vi "Read decimation factors.vi"(8 "error in (no error)":errorcluster, 11 "Runtime.Transfer in":refnum<class "Runtime.Transfer.lvclass">) -> (0 "error out":errorcluster, 2 "decimation factors":T1, 3 "Runtime.Transfer out":refnum<class "Runtime.Transfer.lvclass">)   [LabVIEW 2016, in "Data Sharing Framework.Runtime.lvlib" / "Runtime.Transfer.lvclass"]
uses:
  Runtime.Transfer.lvclass
  Typedefs/Decimation Factors.ctl
  Runtime.Transfer.lvclass/Runtime.Transfer.ctl
  Data Sharing Framework.Configuration.lvlib
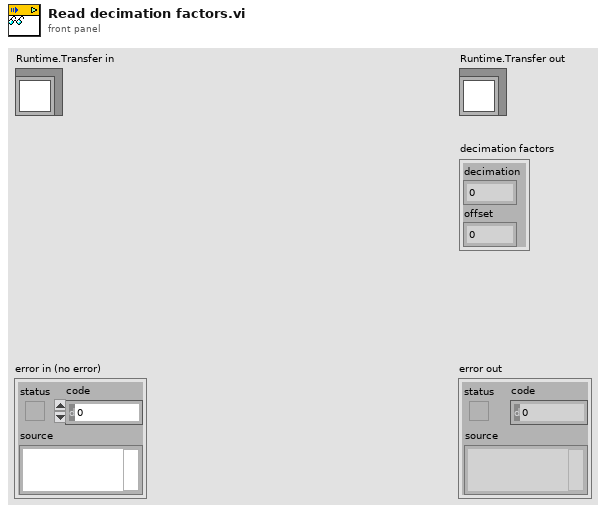
[diagram p1: front panel]
types:
  T1 = typedef "Data Sharing Framework.Configuration.lvlib/Decimation Factors.ctl" = cluster{"decimation":u16, "offset":u16}
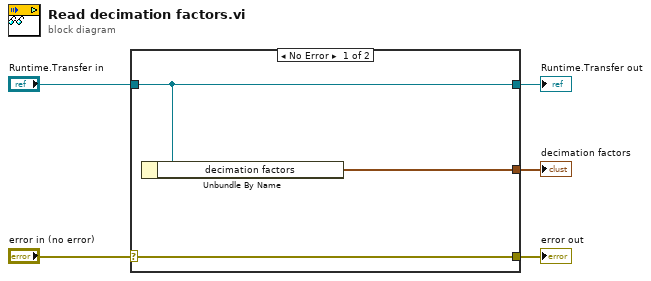
[diagram p0: block diagram]
diagram:
  n1 = case shown="No Error" "error in (no error)" {
    selector: "error in (no error)" -> [w8 w9]
    tunnel: [w8 w9] -> w4
    tunnel: [w7 w10] -> w2
    tunnel: "Runtime.Transfer in" -> [w7 w10]
    tunnel: [w6 _] -> w1
    frame No Error {
      n2 = Unbundle By Name(w7) -> ("decimation factors"=w6:T1)
    }
    frame Error {
    }
  }
  "error out" <- w4
  "Runtime.Transfer out" <- w2
  "decimation factors" <- w1
